vi "Set Up Clock Discipline.vi"(8 "error in (no error)":errorcluster, 11 "RT Data Cluster in":T1={"Timekeeper hdl"="", "clkDisc session"=variant, "Compiled Data"={"SyncMod?"=FALSE, "SyncMod"="", "ConnectionSettings"={"Mode"=enum."Generate sample clock", "pxitrig"=FALSE, "pfi0"=FALSE, "pfi1"=FALSE, "pfi2"=FALSE, "External Pin"=enum."PFI0", "Routes"=[]}, "TimeKeeper"="", "ScanOffset(%)"=0.0, "StartDelay(s)"=0, "Time Ref Settings"={"Time Reference"=enum."GPS", "Priority 1"=0, "Priority 2"=0, "IRIG type"=enum."IRIGB AM", "Terminal"="", "PPSSetTime"=FALSE, "Start Time"=timestamp(0 s since 1904-01-01)}, "FIFO Locations"={"SysTime"=[], "TimeRef"=[], "Status"=[]}}, "OutputsData"=[], "OutputsFIFO"=refnum, "Scan Period"=0, "Timekeeper type"=enum."6683", "SyncMod type"=enum."6683", "SyncMod hdl"=""} {"Compiled Data"."Time Ref Settings"."Priority 2" min=0 max=255; "Compiled Data"."Time Ref Settings"."Priority 1" min=0 max=255}) -> (0 "error out":errorcluster, 3 "RT Data Cluster out":T1={"Timekeeper hdl"="", "clkDisc session"=variant, "Compiled Data"={"SyncMod?"=FALSE, "SyncMod"="", "ConnectionSettings"={"Mode"=enum."Generate sample clock", "pxitrig"=FALSE, "pfi0"=FALSE, "pfi1"=FALSE, "pfi2"=FALSE, "External Pin"=enum."PFI0", "Routes"=[]}, "TimeKeeper"="", "ScanOffset(%)"=0.0, "StartDelay(s)"=0, "Time Ref Settings"={"Time Reference"=enum."GPS", "Priority 1"=0, "Priority 2"=0, "IRIG type"=enum."IRIGB AM", "Terminal"="", "PPSSetTime"=FALSE, "Start Time"=timestamp(0 s since 1904-01-01)}, "FIFO Locations"={"SysTime"=[], "TimeRef"=[], "Status"=[]}}, "OutputsData"=[], "OutputsFIFO"=refnum, "Scan Period"=0, "Timekeeper type"=enum."6683", "SyncMod type"=enum."6683", "SyncMod hdl"=""} {"Compiled Data"."Time Ref Settings"."Priority 2" min=0 max=255; "Compiled Data"."Time Ref Settings"."Priority 1" min=0 max=255})   [LabVIEW 2018, in "Chassis TimeSync Engine.lvlib"]
uses:
  Chassis TimeSync Engine.lvlib
  RT Data Cluster.ctl
  mdevClkDisc.llb/_clkDisc_session.ctl
  Shared/Compiled Data.ctl
  Shared/Connection Settings.ctl
  Shared/Mode.ctl
  Shared/External Pin.ctl
  Shared/Routes.ctl
  Shared/Route.ctl
  Shared/Time Ref Settings.ctl
  Shared/Time Reference.ctl
  Shared/IRIG Type.ctl
  timekeeper type.ctl
  Timekeeper Route Pin.ctl
  <instrlib>/niSync/niSync.llb/niSync Initialize (Default).vi
  Shared/Chassis TimeSync Shared.lvlib
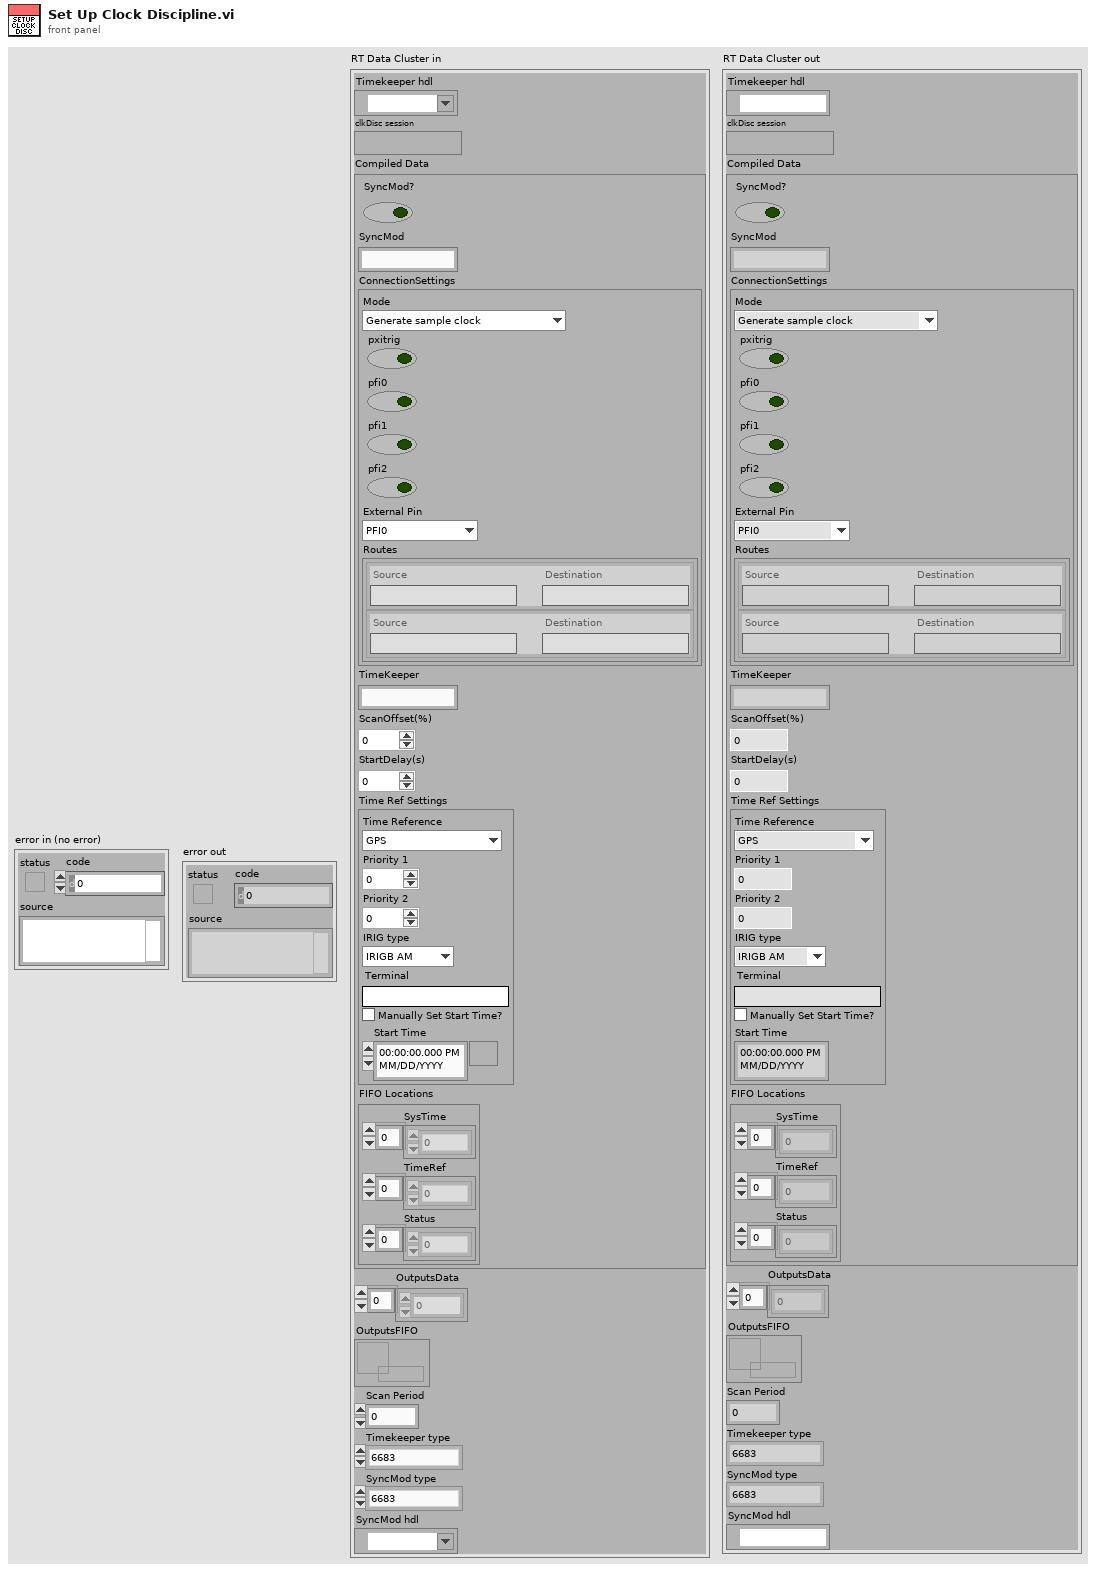
[diagram p1: front panel]
types:
  T1 = typedef "Chassis TimeSync Engine.lvlib/RT Data Cluster.ctl" = cluster{"Timekeeper hdl":refnum<k15>, "clkDisc session":T2, "Compiled Data":T3, "OutputsData":dbl[], "OutputsFIFO":refnum<k33>, "Scan Period":u32, "Timekeeper type":T12, "SyncMod type":T12, "SyncMod hdl":refnum<k15>}
  T2 = typedef "_clkDisc_session.ctl" = variant
  T3 = typedef "Chassis TimeSync Shared.lvlib/Compiled Data.ctl" = cluster{"SyncMod?":bool, "SyncMod":string, "ConnectionSettings":T4, "TimeKeeper":string, "ScanOffset(%)":dbl, "StartDelay(s)":u16, "Time Ref Settings":T9, "FIFO Locations":cluster{"SysTime":i32[], "TimeRef":i32[], "Status":i32[]}}
  T4 = typedef "Chassis TimeSync Shared.lvlib/Connection Settings.ctl" = cluster{"Mode":T5, "pxitrig":bool, "pfi0":bool, "pfi1":bool, "pfi2":bool, "External Pin":T6, "Routes":T7}
  T5 = typedef "Chassis TimeSync Shared.lvlib/Mode.ctl" = enum16{"Generate sample clock", "Route sample clock out of chassis", "Route sample clock into chassis", "Custom routes"}
  T6 = typedef "Chassis TimeSync Shared.lvlib/External Pin.ctl" = enum16{"PFI0", "PFI1", "PFI2"}
  T7 = typedef "Chassis TimeSync Shared.lvlib/Routes.ctl" = T8[]
  T8 = typedef "Chassis TimeSync Shared.lvlib/Route.ctl" = cluster{"Source":string, "Destination":string}
  T9 = typedef "Chassis TimeSync Shared.lvlib/Time Ref Settings.ctl" = cluster{"Time Reference":T10, "Priority 1":i32, "Priority 2":i32, "IRIG type":T11, "Terminal":string, "PPSSetTime":bool, "Start Time":timestamp}
  T10 = typedef "Chassis TimeSync Shared.lvlib/Time Reference.ctl" = enum16{"GPS", "IRIG", "PPS", "1588 Ordinary Clock", "PXI Chassis Clock", "Free Running (Internal)"}
  T11 = typedef "Chassis TimeSync Shared.lvlib/IRIG Type.ctl" = enum16{"IRIGB DC", "IRIGB AM"}
  T12 = typedef "Chassis TimeSync Engine.lvlib/timekeeper type.ctl" = enum16{"6683", "6683H", "6682", "6682H", "non-timekeeper", "timekeeper"}
  T13 = typedef "Chassis TimeSync Engine.lvlib/Timekeeper Route Pin.ctl" = enum16{"TTL0", "PFI0", "PFI1", "PFI2", "PXI_Clk10", "PXI_Clk10_In", "BoardClk", "ClkOut", "Oscillator"}
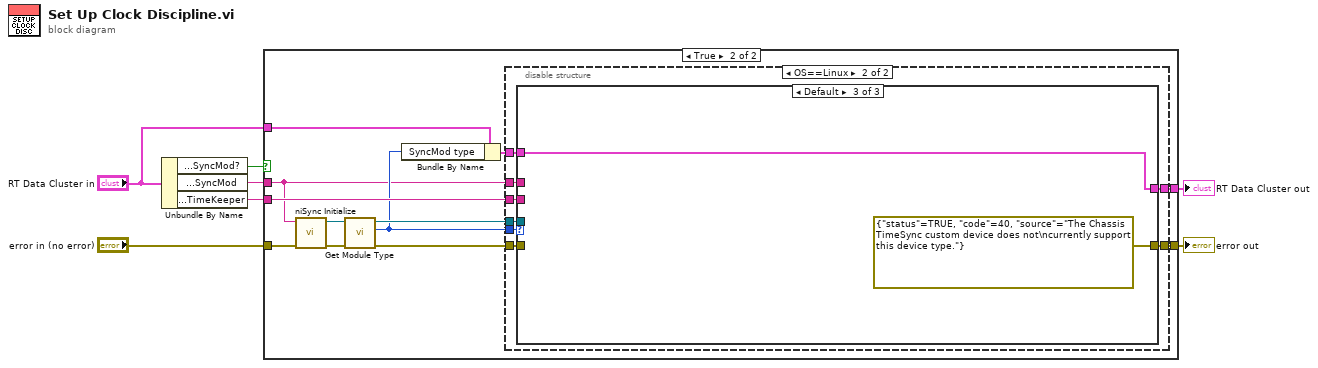
[diagram p0: block diagram]
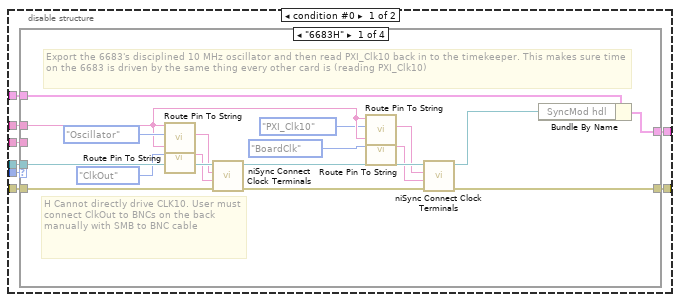
[diagram p3: hidden frame]
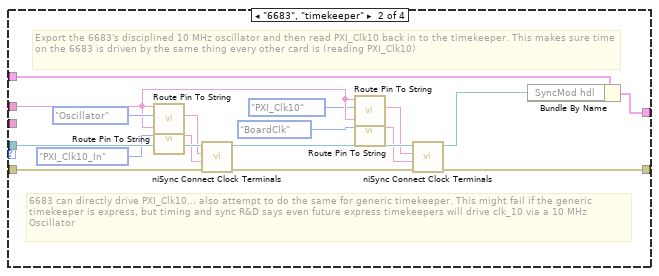
[diagram p4: hidden frame]
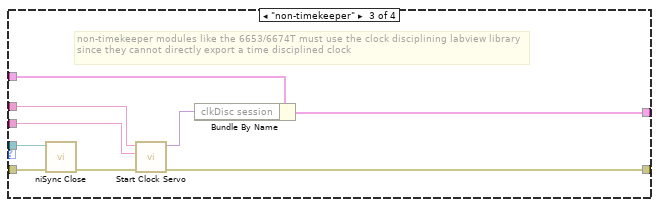
[diagram p5: hidden frame]
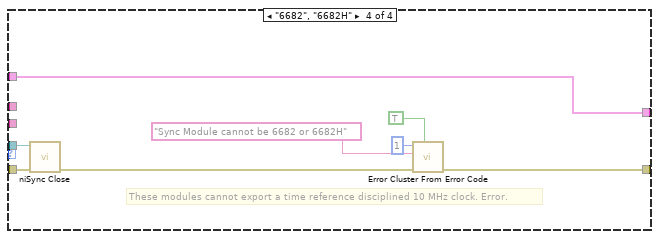
[diagram p6: hidden frame]
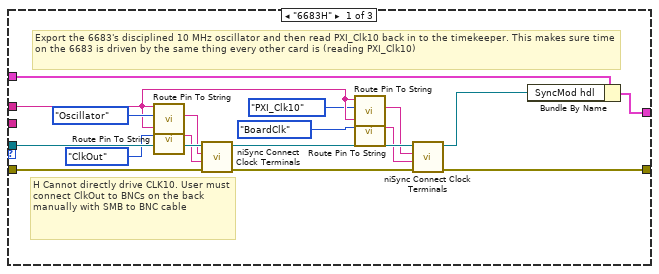
[diagram p7: hidden frame]
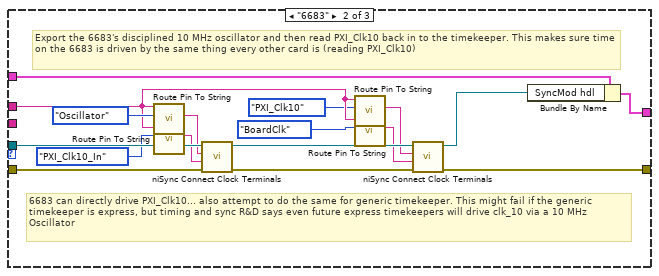
[diagram p8: hidden frame]
diagram:
  n1 = Unbundle By Name("RT Data Cluster in") -> ("Compiled Data.SyncMod?"=w7:bool, "Compiled Data.SyncMod"=w2:string, "Compiled Data.TimeKeeper"=w6:string)
  n2 = case shown="True" w7 {
    tunnel: "error in (no error)" -> [w8 w15]
    tunnel: w6 -> [_ w21]
    tunnel: w2 -> [_ w10]
    tunnel: [w8 w20] -> w5
    tunnel: "RT Data Cluster in" -> [w9 w19]
    tunnel: [w9 w18] -> w3
    frame False {
    }
    frame True {
      n3 = call-poly <instrlib>:"niSync Initialize.vi"("error in (no error)"=w15, "resource name"=w10) -> ("error out"=w17:errorcluster, "instrument handle out"=w16:refnum<k15>)  [unwired: 8 in]
      n4 = call "Get Module Type.vi"("error in (no error)"=w17, "IVI Refnum in"=w16) -> ("error out"=w14:errorcluster, "Module type"=w11:T12, "IVI Refnum out"=w13:refnum<k15>)  [unwired: 6 in, 1 out]
      n5 = Bundle By Name(cluster=w19, "SyncMod type"=w11) -> (w12:T1)
      n6 = disable-structure shown="OS==Linux" {
        disable-tunnel: w21 -> [w29 w88]
        disable-tunnel: [w28 w87] -> w20
        disable-tunnel: [w27 w86] -> w18
        disable-tunnel: w14 -> [w26 w85]
        disable-tunnel: w13 -> [w25 w84]
        disable-tunnel: w12 -> [w24 w83]
        disable-tunnel: w11 -> [w23 w82]
        disable-tunnel: w10 -> [w22 w81]
        frame condition #0 {
          n7 = case shown="\"6683H\"" w23 {
            tunnel: w29 -> [_ _ w72 _]
            tunnel: w22 -> [w32 w49 w71 _]
            tunnel: [w33 w50 w70 w76] -> w28
            tunnel: w24 -> [w46 w63 w69 w75]
            tunnel: [w43 w60 w67 w75] -> w27
            tunnel: w26 -> [w45 w62 w66 w80]
            tunnel: w25 -> [w44 w61 w65 w73]
            frame "6683H" {
              # "Export the 6683's disciplined 10 MHz oscillator and then read PXI_Clk10 back in to the timekeeper. This makes sure time on the 6683 is driven by the same thing every other card is (reading PXI_Clk10)"
              # "H Cannot directly drive CLK10. User must connect ClkOut to BNCs on the back manually with SMB to BNC cable"
              n8 = call "Route Pin To String.vi"("Pin"=Timekeeper_Route_Pin."Oscillator", "Module"=w32) -> ("String"=w42:string)  [unwired: 9 in]
              n9 = call "Route Pin To String.vi"("Pin"=Timekeeper_Route_Pin."ClkOut", "Module"=w32) -> ("String"=w41:string)  [unwired: 9 in]
              n10 = call <instrlib>:"niSync Connect Clock Terminals.vi"("error in (no error)"=w45, "destination terminal"=w41, "source terminal"=w42, "instrument handle"=w44) -> ("error out"=w37:errorcluster, "instrument handle out"=w38:refnum<k15>)  [unwired: 6 in]
              n11 = call "Route Pin To String.vi"("Pin"=Timekeeper_Route_Pin."PXI_Clk10", "Module"=w32) -> ("String"=w35:string)  [unwired: 9 in]
              n12 = call "Route Pin To String.vi"("Pin"=Timekeeper_Route_Pin."BoardClk", "Module"=w32) -> ("String"=w36:string)  [unwired: 9 in]
              n13 = call <instrlib>:"niSync Connect Clock Terminals.vi"("error in (no error)"=w37, "destination terminal"=w36, "source terminal"=w35, "instrument handle"=w38) -> ("error out"=w33:errorcluster, "instrument handle out"=w34:refnum<k15>)  [unwired: 6 in]
              n14 = Bundle By Name(cluster=w46, "SyncMod hdl"=w34) -> (w43:T1)
            }
            frame "6683", "timekeeper" {
              # "6683 can directly drive PXI_Clk10... also attempt to do the same for generic timekeeper. This might fail if the generic timekeeper is express, but timing and sync R&D says even future express timekeepers will drive clk_10 via a 10 MHz Oscillator"
              # "Export the 6683's disciplined 10 MHz oscillator and then read PXI_Clk10 back in to the timekeeper. This makes sure time on the 6683 is driven by the same thing every other card is (reading PXI_Clk10)"
              n15 = call "Route Pin To String.vi"("Pin"=Timekeeper_Route_Pin."Oscillator", "Module"=w49) -> ("String"=w59:string)  [unwired: 9 in]
              n16 = call "Route Pin To String.vi"("Pin"=Timekeeper_Route_Pin."PXI_Clk10_In", "Module"=w49) -> ("String"=w58:string)  [unwired: 9 in]
              n17 = call <instrlib>:"niSync Connect Clock Terminals.vi"("error in (no error)"=w62, "destination terminal"=w58, "source terminal"=w59, "instrument handle"=w61) -> ("error out"=w54:errorcluster, "instrument handle out"=w55:refnum<k15>)  [unwired: 6 in]
              n18 = call "Route Pin To String.vi"("Pin"=Timekeeper_Route_Pin."PXI_Clk10", "Module"=w49) -> ("String"=w52:string)  [unwired: 9 in]
              n19 = call "Route Pin To String.vi"("Pin"=Timekeeper_Route_Pin."BoardClk", "Module"=w49) -> ("String"=w53:string)  [unwired: 9 in]
              n20 = call <instrlib>:"niSync Connect Clock Terminals.vi"("error in (no error)"=w54, "destination terminal"=w53, "source terminal"=w52, "instrument handle"=w55) -> ("error out"=w50:errorcluster, "instrument handle out"=w51:refnum<k15>)  [unwired: 6 in]
              n21 = Bundle By Name(cluster=w63, "SyncMod hdl"=w51) -> (w60:T1)
            }
            frame "non-timekeeper" {
              # "non-timekeeper modules like the 6653/6674T must use the clock disciplining labview library since they cannot directly export a time disciplined clock"
              n22 = call <instrlib>:"niSync Close.vi"("error in (no error)"=w66, "instrument handle"=w65) -> ("error out"=w64:errorcluster)  [unwired: 9 in]
              n23 = call "Start Clock Servo.vi"("error (in)"=w64, "Time-Based Synchronization Module"=w72, "System Timing Module"=w71) -> ("error (out)"=w70:errorcluster, "clkDisc session (out)"=w68:T2)  [unwired: 3 in]
              n24 = Bundle By Name(cluster=w69, "clkDisc session"=w68) -> (w67:T1)
            }
            frame "6682", "6682H" {
              # "These modules cannot export a time reference disciplined 10 MHz clock. Error."
              n25 = call <instrlib>:"niSync Close.vi"("error in (no error)"=w80, "instrument handle"=w73) -> ("error out"=w74:errorcluster)  [unwired: 9 in]
              n26 = call <vilib>:"Error Cluster From Error Code.vi"("show call chain? (False)"=TRUE, "error in (no error)"=w74, "error message (\"\")"="Sync Module cannot be 6682 or 6682H" ("error message (\"\")"), "error code (0)"=1) -> ("error out"=w76:errorcluster)  [unwired: 5 in]
            }
          }
        }
        frame condition #1 (active) {
          n27 = case shown="Default" w82 {
            tunnel: w88 -> [_ _ _]
            tunnel: w81 -> [w91 w108 _]
            tunnel: [w92 w109 errorcluster {"status"=TRUE, "code"=40, "source"="The Chassis TimeSync custom device does not\ncurrently support this device type."} ("error out")] -> w87
            tunnel: w83 -> [w105 w122 w124]
            tunnel: [w102 w119 w124] -> w86
            tunnel: w85 -> [w104 w121 _]
            tunnel: w84 -> [w103 w120 _]
            frame "6683H" {
              # "Export the 6683's disciplined 10 MHz oscillator and then read PXI_Clk10 back in to the timekeeper. This makes sure time on the 6683 is driven by the same thing every other card is (reading PXI_Clk10)"
              # "H Cannot directly drive CLK10. User must connect ClkOut to BNCs on the back manually with SMB to BNC cable"
              n28 = call "Route Pin To String.vi"("Pin"=Timekeeper_Route_Pin."Oscillator", "Module"=w91) -> ("String"=w101:string)  [unwired: 9 in]
              n29 = call "Route Pin To String.vi"("Pin"=Timekeeper_Route_Pin."ClkOut", "Module"=w91) -> ("String"=w100:string)  [unwired: 9 in]
              n30 = call <instrlib>:"niSync Connect Clock Terminals.vi"("error in (no error)"=w104, "destination terminal"=w100, "source terminal"=w101, "instrument handle"=w103) -> ("error out"=w96:errorcluster, "instrument handle out"=w97:refnum<k15>)  [unwired: 6 in]
              n31 = call "Route Pin To String.vi"("Pin"=Timekeeper_Route_Pin."PXI_Clk10", "Module"=w91) -> ("String"=w94:string)  [unwired: 9 in]
              n32 = call "Route Pin To String.vi"("Pin"=Timekeeper_Route_Pin."BoardClk", "Module"=w91) -> ("String"=w95:string)  [unwired: 9 in]
              n33 = call <instrlib>:"niSync Connect Clock Terminals.vi"("error in (no error)"=w96, "destination terminal"=w95, "source terminal"=w94, "instrument handle"=w97) -> ("error out"=w92:errorcluster, "instrument handle out"=w93:refnum<k15>)  [unwired: 6 in]
              n34 = Bundle By Name(cluster=w105, "SyncMod hdl"=w93) -> (w102:T1)
            }
            frame "6683" {
              # "6683 can directly drive PXI_Clk10... also attempt to do the same for generic timekeeper. This might fail if the generic timekeeper is express, but timing and sync R&D says even future express timekeepers will drive clk_10 via a 10 MHz Oscillator"
              # "Export the 6683's disciplined 10 MHz oscillator and then read PXI_Clk10 back in to the timekeeper. This makes sure time on the 6683 is driven by the same thing every other card is (reading PXI_Clk10)"
              n35 = call "Route Pin To String.vi"("Pin"=Timekeeper_Route_Pin."Oscillator", "Module"=w108) -> ("String"=w118:string)  [unwired: 9 in]
              n36 = call "Route Pin To String.vi"("Pin"=Timekeeper_Route_Pin."PXI_Clk10_In", "Module"=w108) -> ("String"=w117:string)  [unwired: 9 in]
              n37 = call <instrlib>:"niSync Connect Clock Terminals.vi"("error in (no error)"=w121, "destination terminal"=w117, "source terminal"=w118, "instrument handle"=w120) -> ("error out"=w113:errorcluster, "instrument handle out"=w114:refnum<k15>)  [unwired: 6 in]
              n38 = call "Route Pin To String.vi"("Pin"=Timekeeper_Route_Pin."PXI_Clk10", "Module"=w108) -> ("String"=w111:string)  [unwired: 9 in]
              n39 = call "Route Pin To String.vi"("Pin"=Timekeeper_Route_Pin."BoardClk", "Module"=w108) -> ("String"=w112:string)  [unwired: 9 in]
              n40 = call <instrlib>:"niSync Connect Clock Terminals.vi"("error in (no error)"=w113, "destination terminal"=w112, "source terminal"=w111, "instrument handle"=w114) -> ("error out"=w109:errorcluster, "instrument handle out"=w110:refnum<k15>)  [unwired: 6 in]
              n41 = Bundle By Name(cluster=w122, "SyncMod hdl"=w110) -> (w119:T1)
            }
            frame Default {
            }
          }
        }
      }
    }
  }
  "error out" <- w5
  "RT Data Cluster out" <- w3
